vi "THzTimeScan_830.vi"(0 "input":T1) -> (1 "loop stop":bool, 2 "x-axis":sgl[](array[numeric]), 3 "y-axis":dbl[](array[numeric]))   [LabVIEW 2010]
uses:
  <vilib>/Utility/file.llb/Write To Spreadsheet File (string).vi
panel:
  out "Current Position":dbl
  out "Array":dbl[](array[numeric])
  out "String":string
  out "Read position":bool
  out "Ask position":bool
  out "Move delay":bool
  out "Read830":bool
  out "Command":string
  out "THz Signal Graph":dbl(graph)
  in  "loop stop":bool
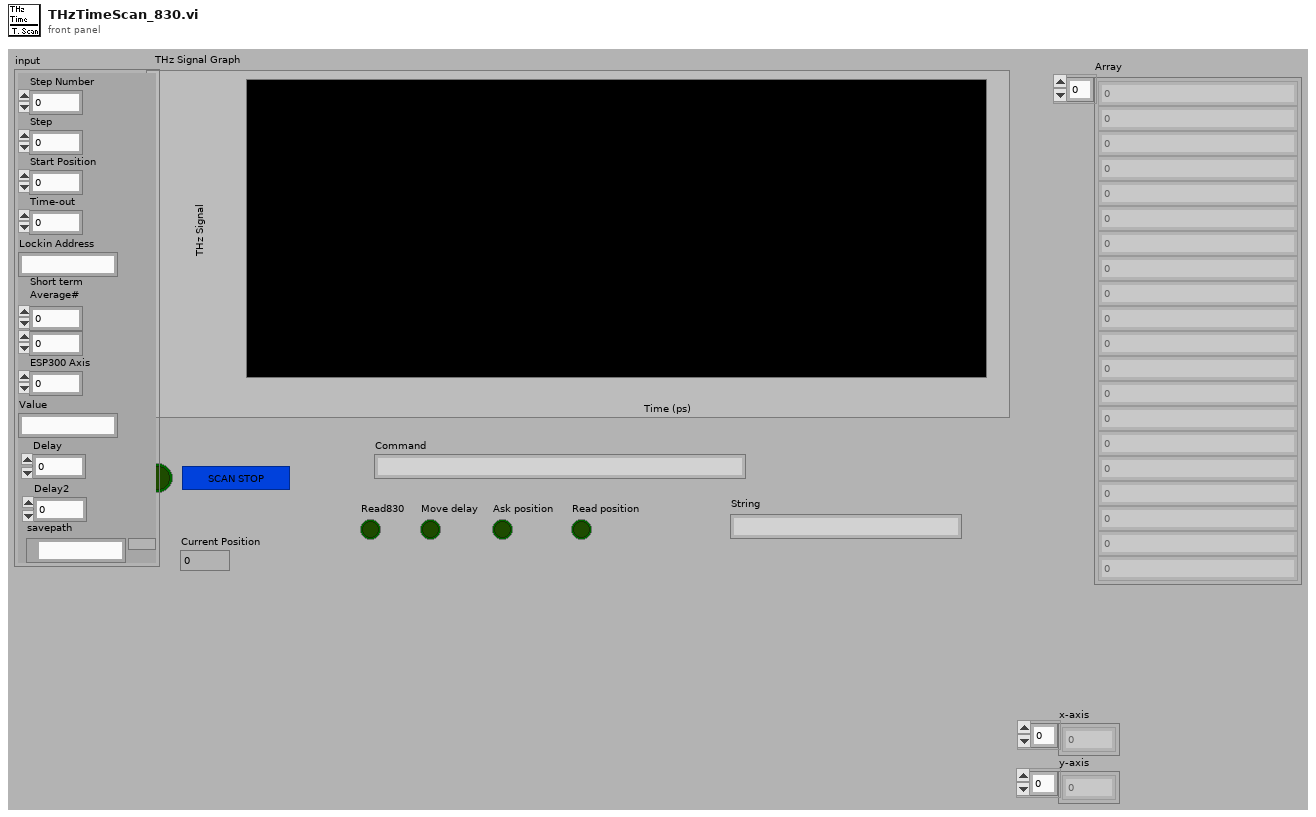
[diagram p1: front panel]
types:
  T1 = cluster{"Step Number":i32, "Step":sgl, "Start Position":sgl, "Time-out":i32, "Lockin Address":string, "Short term \nAverage#":i8, i32, "ESP300 Axis":i8, "Value":string, "Delay":dbl, "Delay2":dbl, "savepath":path}
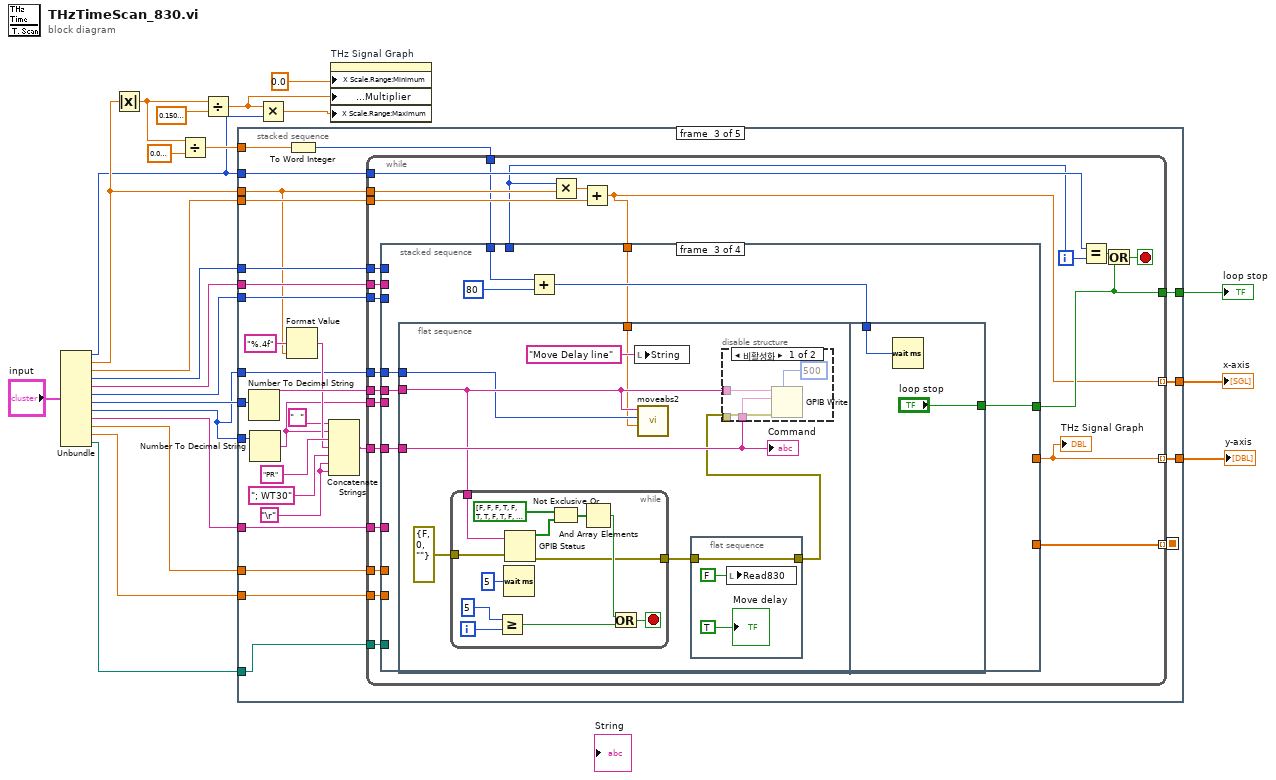
[diagram p0: block diagram]
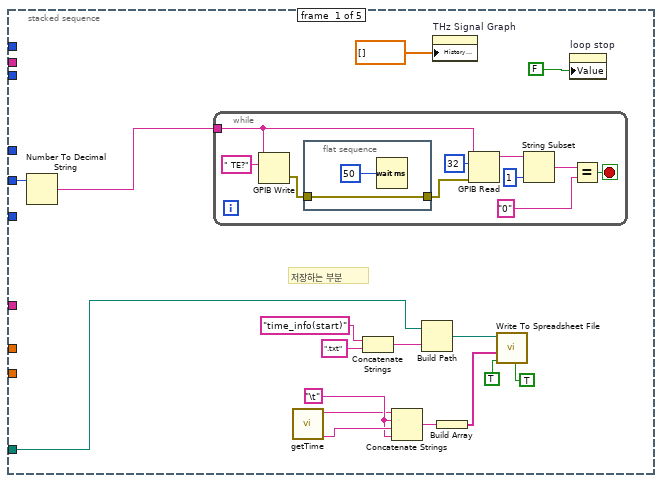
[diagram p2: hidden frame]
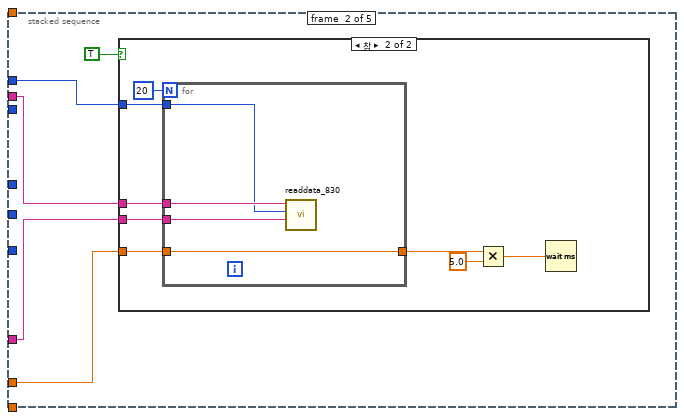
[diagram p3: hidden frame]
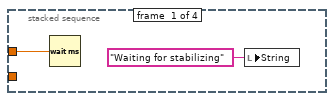
[diagram p5: hidden frame]
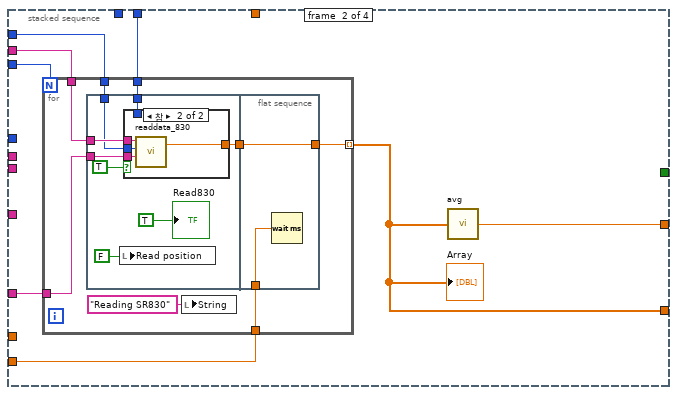
[diagram p6: hidden frame]
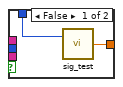
[diagram p7: hidden frame]
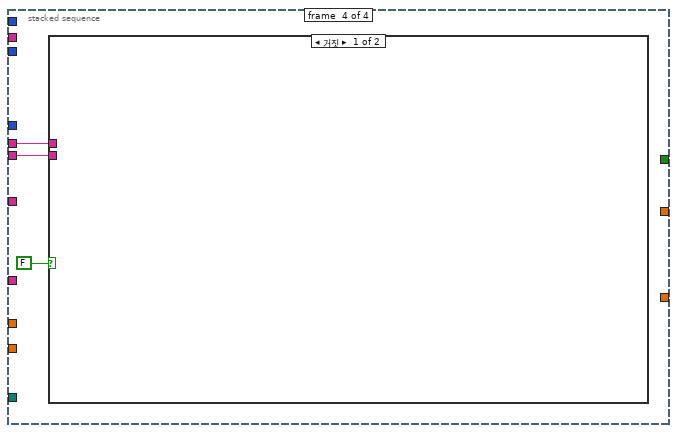
[diagram p9: hidden frame]
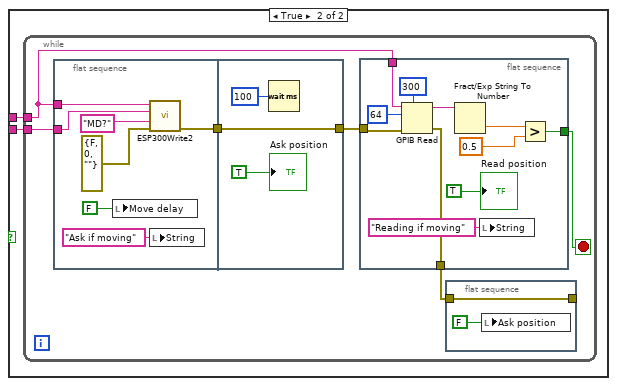
[diagram p10: hidden frame]
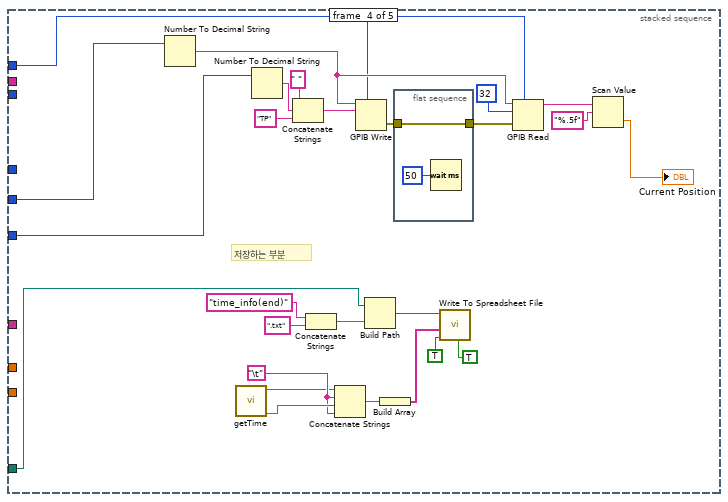
[diagram p11: hidden frame]
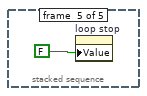
[diagram p12: hidden frame]
diagram:
  n1 = Unbundle("input") -> ("Step Number"=w9:i32, "Step"=w15:sgl, "Start Position"=w14:sgl, "Time-out"=w13:i32, "Lockin Address"=w12:string, "Short term \nAverage#"=w5:i8, w11:i32, "ESP300 Axis"=w1:i8, "Value"=w10:string, "Delay"=w4:dbl, "Delay2"=w3:dbl, "savepath"=w2:path)
  n2 = Absolute Value(x=w15) -> (abs(x)=w19:sgl)
  n3 = Divide(x=w19, y=sgl 0.004) -> (x/y=w17:sgl)
  n4 = Divide(x=w19, y=sgl 0.15) -> (x/y=w7:sgl)
  n5 = stacked-sequence {
    seq-local: [_ _ w72 _ _] -> [_ _ _ _ _]
    tunnel: w14 -> [_ _ w96 _ _]
    tunnel: w13 -> [_ w56 w95 w225 _]
    tunnel: w12 -> [_ w55 w94 _ _]
    tunnel: w5 -> [_ _ w93 _ _]
    tunnel: w11 -> [w37 _ w88 w227 _]
    tunnel: w1 -> [_ _ w86 w228 _]
    tunnel: w10 -> [_ w54 w78 _ _]
    tunnel: [_ _ w92 _ _] -> w23
    tunnel: [_ _ w91 _ _] -> w22
    tunnel: [_ _ w90 _ _] -> w21
    tunnel: w15 -> [_ _ w84 _ _]
    tunnel: w9 -> [_ _ w89 _ _]
    tunnel: w17 -> [_ _ w83 _ _]
    tunnel: w4 -> [_ w52 w74 _ _]
    tunnel: w3 -> [_ _ w73 _ _]
    tunnel: w2 -> [w24 _ w70 w239 _]
    tunnel: w1 -> [_ _ w69 _ _]
    frame #0 {
      w27 = "\t"
      # "저장하는 부분"
      n6 = Number To Decimal String(number=w37) -> (decimal integer string=w36:string)  [unwired: 1 in]
      n7 = while {
        tunnel: w36 -> [w42]
        stop <- w47 stop-if-true
        n8 = GPIB Write(0:w42, 1:" TE?" ("data")) -> (6:w41:errorcluster)  [unwired: 3 in, 1 out]
        n9 = flat-sequence {
          tunnel: w41 -> [w51]
          tunnel: [w51] -> w40
          frame #0 {
            n10 = Wait (ms)(milliseconds to wait=u32 50) -> ()  [unwired: 1 out]
          }
        }
        n11 = GPIB Read(0:w42, 1:32 ("byte count"), 3:w40) -> (5:w46:string)  [unwired: 2 in, 2 out]
        n12 = String Subset(string=w46, length (rest)=1 ("offset (0)")) -> (substring=w44:string)  [unwired: 1 in]
        n13 = Equal?(x=w44, y="0") -> (x = y?=w47:bool)
      }
      n14 = call "getTime.vi"() -> ("시간"=w28:string, "날짜"=w26:string)  [unwired: 10 in]
      n15 = Concatenate Strings("time_info(start)" ("string"), ".txt" ("string")) -> (w34:string)
      n16 = Concatenate Strings(w26, w27, w28, w27) -> (w25:string)
      n17 = Build Path(base path=w24, name or relative path=w34) -> (appended path=w31:path)
      n18 = property on="THz Signal Graph" class="WFChart (엄격한)"("History Data"=dbl[] []) -> ()  [unwired: 2 in, 2 out]
      n19 = Build Array(w25) -> (w30:string[])
      n20 = call-poly <vilib>:"Write To Spreadsheet File.vi"("transpose? (no:F)"=TRUE ("transpose?\n(no:F)"), "append to file? (new file:F)"=TRUE ("transpose?\n(no:F)"), "1D data"=w30, "file path (dialog if empty)"=w31) -> ()  [unwired: 4 in, 1 out]
      n21 = property on="loop stop" class="Bool (엄격한)"("Value"=FALSE) -> ()  [unwired: 2 in, 2 out]
    }
    frame #1 {
      n22 = case shown="참" TRUE {
        tunnel: w56 -> [_ w63]
        tunnel: w55 -> [_ w62]
        tunnel: w54 -> [_ w61]
        tunnel: w52 -> [_ w60]
        frame False {
        }
        frame True {
          n23 = for {
            N: 20 -> [_]
            tunnel: w62 -> [w68]
            tunnel: w61 -> [w67]
            tunnel: w63 -> [w66]
            tunnel: w60 -> [w65]
            tunnel: [w65] -> w59
            n24 = call "readdata_830.vi"("Command"=w67, "timeout"=w66, "Lockin Address"=w68) -> ()  [unwired: 1 in, 2 out]
          }
          n25 = Multiply(x=w59, y=5.0) -> (x*y=w57:dbl)
          n26 = Wait (ms)(milliseconds to wait=w57) -> ()  [unwired: 1 out]
        }
      }
    }
    frame #2 {
      w77 = "\r"
      n27 = Number To Decimal String(number=w88) -> (decimal integer string=w87:string)  [unwired: 1 in]
      n28 = Number To Decimal String(number=w86) -> (decimal integer string=w75:string)  [unwired: 1 in]
      n29 = Format Value(format string="%.4f", value (0)=w84) -> (output string=w80:string)  [unwired: 1 in]
      n30 = To Word Integer(number=w83) -> (16bit integer=w82:i16)
      n31 = Concatenate Strings("  " ("string"), w75, "PR" ("Substring"), w80, "; WT30" ("string"), w77, w77) -> (w71:string)
      n32 = while {
        tunnel: [w105] -> w92
        tunnel: [w111] -> w90 mode=indexing
        tunnel: [w97] -> w91 mode=indexing
        tunnel: w89 -> [w116]
        tunnel: w84 -> [w115]
        tunnel: w96 -> [w114]
        tunnel: w95 -> [w106]
        tunnel: w94 -> [w113]
        tunnel: w93 -> [w112]
        tunnel: w87 -> [w110]
        tunnel: w71 -> [w109]
        tunnel: w82 -> [w108]
        tunnel: w78 -> [w107]
        tunnel: w75 -> [w104]
        tunnel: w74 -> [w103]
        tunnel: w73 -> [w102]
        tunnel: [w101] -> w72 mode=indexing
        tunnel: w70 -> [w99]
        tunnel: w69 -> [w98]
        i -> [w100]
        stop <- w119 stop-if-true
        n33 = Multiply(x=w100, y=w115) -> (x*y=w117:sgl)
        n34 = Add(x=w117, y=w114) -> (x+y=w97:sgl)
        n35 = stacked-sequence {
          tunnel: w113 -> [_ w126 _ _]
          tunnel: [_ w128 _ _] -> w111
          tunnel: w112 -> [_ w129 _ _]
          tunnel: w110 -> [_ _ w160 w193]
          tunnel: w109 -> [_ _ w161 _]
          tunnel: w108 -> [_ _ w159 _]
          tunnel: w107 -> [_ w127 _ _]
          tunnel: w106 -> [_ w125 _ _]
          tunnel: [_ _ w156 _] -> w105
          tunnel: w104 -> [_ _ _ w192]
          tunnel: w103 -> [w121 _ _ _]
          tunnel: w102 -> [_ w124 _ _]
          tunnel: [_ w123 _ _] -> w101
          tunnel: w100 -> [_ w122 _ _]
          tunnel: w99 -> [_ _ _ _]
          tunnel: w98 -> [_ _ w155 _]
          tunnel: w97 -> [_ _ w154 _]
          frame #0 {
            n36 = Wait (ms)(milliseconds to wait=w121) -> ()  [unwired: 1 out]
            n37 = local write "String"("Waiting for stabilizing" ("String")) -> ()
          }
          frame #1 {
            n38 = for {
              N: w129 -> [_]
              tunnel: w126 -> [w134]
              tunnel: w125 -> [w137]
              tunnel: [w136] -> w123 mode=indexing
              tunnel: w127 -> [w135]
              tunnel: w124 -> [w131]
              tunnel: w122 -> [w130]
              n39 = flat-sequence {
                tunnel: w137 -> [w141]
                tunnel: w135 -> [w142]
                tunnel: w134 -> [w143]
                tunnel: [w140] -> w132
                tunnel: w130 -> [w138]
                tunnel: [w153] -> w136
                tunnel: w132 -> [w153]
                tunnel: w131 -> [w152]
                frame #0 {
                  n40 = local write "Read position"(FALSE ("Read position")) -> ()
                  n41 = case shown="참" TRUE {
                    tunnel: w143 -> [_ w151]
                    tunnel: w142 -> [_ w150]
                    tunnel: w141 -> [_ w149]
                    tunnel: [w147 w148] -> w140
                    tunnel: w138 -> [w146 _]
                    frame False {
                      n42 = call "sig_test.vi"("index (row)"=w146) -> ("element"=w147:dbl)  [unwired: 1 in]
                    }
                    frame True {
                      n43 = call "readdata_830.vi"("Command"=w150, "timeout"=w149, "Lockin Address"=w151) -> ("Data"=w148:dbl)  [unwired: 1 in, 1 out]
                    }
                  }
                  "Read830" <- TRUE ("Read830")
                }
                frame #1 {
                  n44 = Wait (ms)(milliseconds to wait=w152) -> ()  [unwired: 1 out]
                }
              }
              n45 = local write "String"("Reading SR830" ("String")) -> ()
            }
            "Array" <- w123
            n46 = call "avg.vi"("Array"=w123) -> ("Numeric"=w128:dbl)
          }
          frame #2 {
            n47 = flat-sequence {
              tunnel: w161 -> [w169]
              tunnel: w160 -> [w164]
              tunnel: w155 -> [w163]
              tunnel: w154 -> [w162]
              tunnel: w158 -> [w189]
              tunnel: ["loop stop"] -> w156
              frame #0 {
                n48 = while {
                  tunnel: errorcluster {"status"=FALSE, "code"=0, "source"=""} ("error in (no error)") -> [w188]
                  tunnel: [w178] -> w166
                  tunnel: w164 -> [w177]
                  i -> [w187]
                  stop <- w184 stop-if-true
                  n49 = Greater Or Equal?(x=5, y=w187) -> (x >= y?=w185:bool)
                  n50 = Wait (ms)(milliseconds to wait=u32 5) -> ()  [unwired: 1 out]
                  n51 = GPIB Status(0:w177, 1:w188) -> (2:w182:bool[], 5:w178:errorcluster)  [unwired: 2 out]
                  n52 = Not Exclusive Or(1:w182, 2:bool[] [FALSE, FALSE, FALSE, TRUE, FALSE, TRUE, TRUE, FALSE, TRUE, FALSE, FALSE, FALSE, FALSE, FALSE, FALSE, FALSE] ("status 2")) -> (0:w181:bool[])
                  n53 = And Array Elements(Boolean array=w181) -> (logical AND=w180:bool)
                  n54 = Or(x=w180, y=w185) -> (x .or. y?=w184:bool)
                }
                n55 = local write "String"("Move Delay line" ("String")) -> ()
                n56 = call "moveabs2.vi"("SetPosition"=w162, "EXP300 Axis"=w163, "THz Image\nESP Address"=w164) -> ()  [unwired: 1 in, 1 out]
                n57 = flat-sequence {
                  tunnel: [w176] -> w167
                  tunnel: w166 -> [w176]
                  frame #0 {
                    n58 = local write "Read830"(FALSE ("Read830")) -> ()
                    "Move delay" <- TRUE ("Move delay")
                  }
                }
                n59 = disable-structure shown="비활성화" {
                  disable-tunnel: w169 -> [w173 _]
                  disable-tunnel: w167 -> [w171 _]
                  disable-tunnel: w164 -> [w170 _]
                  frame Disabled {
                    n60 = GPIB Write(0:w170, 1:w173, 3:w171, 4:500 ("timeout ms (488.2 global)")) -> ()  [unwired: 1 in, 2 out]
                  }
                  frame Enabled {
                  }
                }
                "Command" <- w169
              }
              frame #1 {
                n61 = Wait (ms)(milliseconds to wait=w189) -> ()  [unwired: 1 out]
              }
            }
            n62 = Add(x=w159, y=i16 80) -> (x+y=w158:i16)
          }
          frame #3 {
            n63 = case shown="거짓" FALSE {
              tunnel: w193 -> [_ w195]
              tunnel: w192 -> [_ w194]
              frame False {
              }
              frame True {
                n64 = while {
                  tunnel: w195 -> [w197]
                  tunnel: w194 -> [w201]
                  stop <- w199 stop-if-true
                  n65 = flat-sequence {
                    tunnel: w201 -> [w215]
                    tunnel: w197 -> [w218]
                    tunnel: [w219] -> w198
                    tunnel: [w224] -> w200
                    tunnel: w198 -> [w224]
                    frame #0 {
                      n66 = local write "Move delay"(FALSE ("Move delay")) -> ()
                      n67 = call "ESP300Write2.vi"("error in (no error)"=errorcluster {"status"=FALSE, "code"=0, "source"=""}, "Command"="MD?", "ESP300 Channel"=w215, "ESP300 Address"=w218) -> ("error out"=w219:errorcluster)  [unwired: 3 in]
                      n68 = local write "String"("Ask if moving" ("String")) -> ()
                    }
                    frame #1 {
                      n69 = Wait (ms)(milliseconds to wait=u32 100) -> ()  [unwired: 1 out]
                      "Ask position" <- TRUE ("Ask position")
                    }
                  }
                  n70 = flat-sequence {
                    tunnel: w200 -> [w214]
                    tunnel: [w211] -> w199
                    tunnel: w197 -> [w207]
                    tunnel: [w205] -> w196
                    frame #0 {
                      n71 = GPIB Read(0:w207, 1:64 ("byte count"), 3:w214, 4:300 ("timeout ms (488.2 global)")) -> (5:w210:string, 7:w205:errorcluster)  [unwired: 1 in, 1 out]
                      n72 = Fract/Exp String To Number(string=w210) -> (number=w209:dbl)  [unwired: 3 in, 1 out]
                      n73 = local write "String"("Reading if moving" ("String")) -> ()
                      n74 = Greater?(x=w209, y=0.5) -> (0:w211:bool)
                      "Read position" <- TRUE ("Read position")
                    }
                  }
                  n75 = flat-sequence {
                    tunnel: [w203] -> _
                    tunnel: w196 -> [w203]
                    frame #0 {
                      n76 = local write "Ask position"(FALSE ("Ask position")) -> ()
                    }
                  }
                }
              }
            }
          }
        }
        "THz Signal Graph" <- w111
        n77 = Equal?(x=w116, y=w100) -> (x = y?=w118:bool)
        n78 = Or(x=w118, y=w105) -> (x .or. y?=w119:bool)
      }
    }
    frame #3 {
      w242 = "\t"
      # "저장하는 부분"
      n79 = Number To Decimal String(number=w227) -> (decimal integer string=w226:string)  [unwired: 1 in]
      n80 = call "getTime.vi"() -> ("시간"=w243:string, "날짜"=w241:string)  [unwired: 10 in]
      n81 = Number To Decimal String(number=w228) -> (decimal integer string=w230:string)  [unwired: 1 in]
      n82 = Concatenate Strings(" " ("string"), w230, "TP" ("string")) -> (w234:string)
      n83 = Concatenate Strings("time_info(end)" ("string"), ".txt" ("string")) -> (w249:string)
      n84 = Concatenate Strings(w241, w242, w243, w242) -> (w240:string)
      n85 = GPIB Write(0:w226, 1:w234, 4:w225) -> (6:w232:errorcluster)  [unwired: 2 in, 1 out]
      n86 = Build Path(base path=w239, name or relative path=w249) -> (appended path=w246:path)
      n87 = Build Array(w240) -> (w245:string[])
      n88 = flat-sequence {
        tunnel: w232 -> [w252]
        tunnel: [w252] -> w231
        frame #0 {
          n89 = Wait (ms)(milliseconds to wait=u32 50) -> ()  [unwired: 1 out]
        }
      }
      n90 = call-poly <vilib>:"Write To Spreadsheet File.vi"("transpose? (no:F)"=TRUE ("transpose?\n(no:F)"), "append to file? (new file:F)"=TRUE ("transpose?\n(no:F)"), "1D data"=w245, "file path (dialog if empty)"=w246) -> ()  [unwired: 4 in, 1 out]
      n91 = GPIB Read(0:w226, 1:32 ("byte count"), 3:w231, 4:w225) -> (5:w236:string)  [unwired: 1 in, 2 out]
      n92 = Scan Value(string=w236, format string="%.5f") -> (value=→"Current Position":dbl)  [unwired: 1 in, 1 out]
    }
    frame #4 {
      n93 = property on="loop stop" class="Bool (엄격한)"("Value"=FALSE) -> ()  [unwired: 2 in, 2 out]
    }
  }
  "loop stop" <- w23
  "x-axis" <- w22
  "y-axis" <- w21
  n94 = Multiply(x=w7, y=w9) -> (x*y=w6:sgl)
  n95 = property on="THz Signal Graph" class="WFChart (엄격한)"("X Scale.Range:Minimum"=0.0, "X Scale.Offset and Multiplier:Multiplier"=w7, "X Scale.Range:Maximum"=w6) -> ()  [unwired: 2 in, 2 out]
